vi "OFDM-SIM子载波调制.vi"(3 "error in":errorcluster caption="error in (no error)", 4 "并行信号":cdb[][](array[numeric]), 5 "载波数":i32=125, 6 "SIM比特":i32[](array[numeric])) -> (0 "error out":errorcluster, 1 "实际输入序列":i32[](array[numeric]), 2 "SIM输出":cdb[][](array[numeric]))   [LabVIEW 2018]
uses:
  <vilib>/addons/Modulation/Digital/General/MT Generate QAM System Parameters(M).vi
  <vilib>/addons/Modulation/Digital/General/MT Map QAM Symbols to Bits.vi
  <vilib>/addons/Modulation/niDMT.lvlib
panel:
  in  "M-QAM":i32=4 caption="M-QAM (16)"
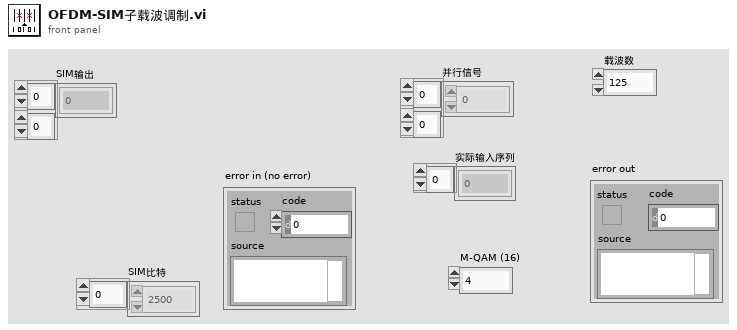
[diagram p1: front panel]
types:
  T1 = cluster{"samples per symbol (16)":i32, "symbol map":cdb[]}
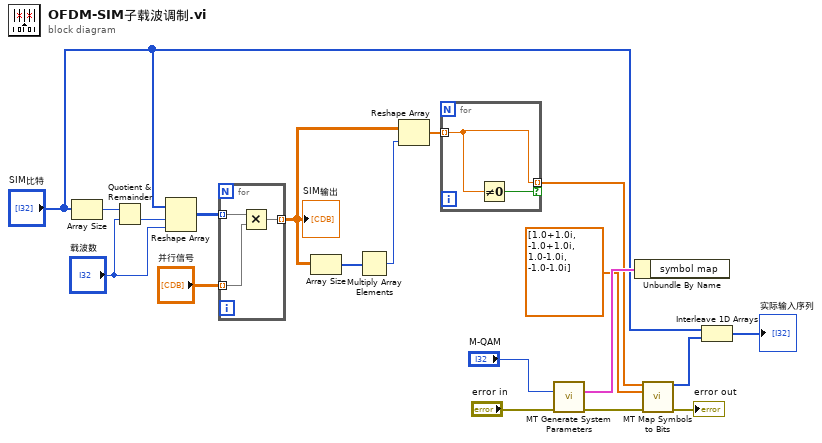
[diagram p0: block diagram]
diagram:
  n1 = Array Size(array="SIM比特") -> (size(s)=w19:i32)
  n2 = Quotient & Remainder(x=w19, y="载波数") -> (floor(x/y)=w18:i32)  [unwired: 1 out]
  n3 = Reshape Array ("重排数组维数")("SIM比特", w18, "载波数") -> (w16:i32[][])
  n4 = for {
    tunnel: w16 -> [w21] mode=indexing
    tunnel: "并行信号" -> [w22] mode=indexing
    tunnel: [w20] -> w8 mode=indexing
    n5 = Multiply(x=w21, y=w22) -> (x*y=w20:cdb[])
  }
  "SIM输出" <- w8
  n6 = Array Size(array=w8) -> (size(s)=w9:i32[])
  n7 = Multiply Array Elements(1:w9) -> (0:w10:i32)
  n8 = Reshape Array(w8, w10) -> (w2:cdb[])
  n9 = for {
    tunnel: w2 -> [w23] mode=indexing
    tunnel: [w23] -> w3 mode=indexing if=w24
    n10 = Not Equal To 0?(x=w23) -> (x != 0?=w24:bool)
  }
  n11 = call-poly <vilib>:"MT Generate System Parameters.vi"("M-QAM (16)"="M-QAM", "error in (no error)"="error in") -> ("QAM system parameters"=w14:T1, "error out"=w12:errorcluster)  [unwired: 11 in, 1 out]
  n12 = Unbundle By Name(w14) -> ()  [unwired: 1 out]
  n13 = call-poly <vilib>:"MT Map Symbols to Bits.vi"("symbols"=w3, "symbol map"=cdb[] [1.0+1.0i, -1.0+1.0i, 1.0-1.0i, -1.0-1.0i], "error in (no error)"=w12) -> ("output bit stream"=w4:i8[], "error out"=→"error out":errorcluster)  [unwired: 11 in]
  n14 = Interleave 1D Arrays("SIM比特", w4) -> (→"实际输入序列":i32[])
